vi "Plot Group Config Prompt.vi"(7 "Manager":refnum<class "MessageQ.lvclass">, 9 "Config in":T1, 10 "Init Available Channels":string[](array[string])) -> (1 "Config":T1, 2 "Cancelled":bool)   [LabVIEW 2020, in "VolatusGUIElements.lvlib" / "HistorianCharting.lvclass"]
uses:
  HistorianCharting.lvclass
  VolatusGUI/Historian Charting Manager/X-Axis Type.ctl
  VolatusGUI/Historian Charting Manager/Plot Group Config.ctl
  VolatusGUI/Historian Charting Manager/Plot Config.ctl
  VolatusGUI/Historian Charting Manager/Scale.ctl
  Volatus/MessageQ/MessageQ.lvclass
  lv-autocomplete/AutoComplete/AutoComplete/AutoComplete.lvclass/AutoComplete.ctl
  Volatus/MessageQ/MessageQ.lvclass/MessageQ.ctl
  f20c74bd-5406-41d2-98d9-ce743746d173.vi
  6165f306-330e-4d21-bc48-f8023b5fd340.vi
  c136c978-185a-46ef-8da4-aa5ceb8485eb.vi
  9b52c319-6332-4e64-8368-05bb343efa0c.vi
  lv-autocomplete/AutoComplete/Launch Autocomplete Handler.vi
  <vilib>/Comparison/Less/Less Functor/Less Functor.lvclass
  lv-autocomplete/AutoComplete/AutoComplete/AutoComplete.lvclass
  <vilib>/Comparison/Equal/Equal Functor/Equal Functor.lvclass
  VolatusGUI/Historian Charting Manager/Historian Charting Manager.lvclass
panel:
  out "Group Changes":bool
  in  "X-Axis List":i32(listbox)
  out "Unselected Channels":string[](array[string])
  in  "Dup Group":bool
  in  "X-Axis Channel":string
  in  "Cancel":bool
  in  "Accept":bool
  in  "X-Axis Type":T2
  in  "Remove Group":bool
  in  "New Group":bool
  out "Plot Group":string
  in  "Clear Filter":bool
  in  "Available Channels":i32(listbox)
  in  "Filter":string
  in  "Selected Channels":i32(listbox)
  # "Available Channels"
  # "Double-click to remove channel\nDrag to reorder"
  # "Double-click to add channel"
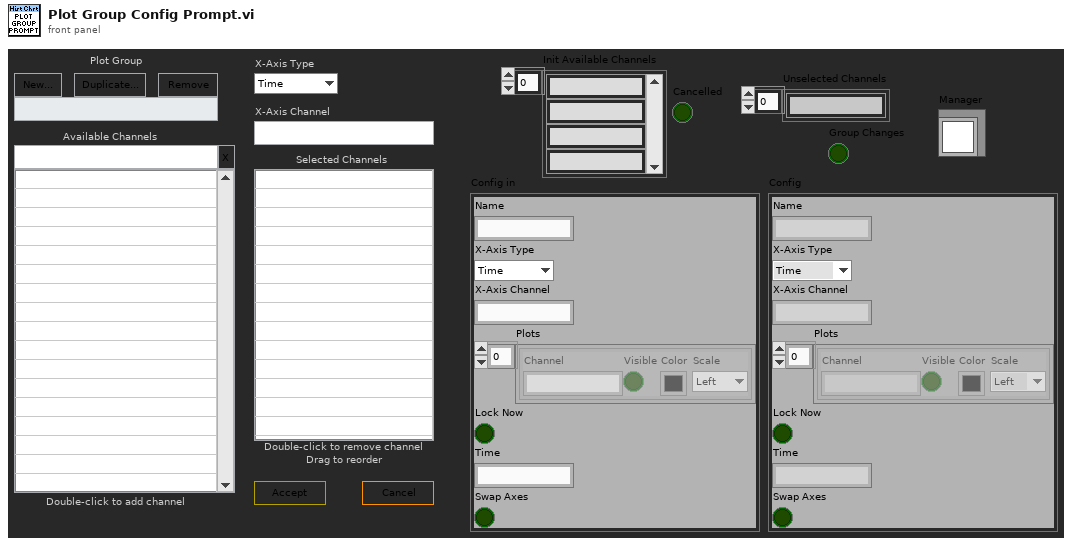
[diagram p1: front panel]
types:
  T1 = typedef "VolatusGUI.lvlib/Historian Charting Manager.lvclass/Plot Group Config.ctl" = cluster{"Name":string, "X-Axis Type":T2, "X-Axis Channel":string, "Plots":T3[], "Lock Now":bool, "Time":string, "Swap Axes":bool}
  T2 = typedef "VolatusGUI.lvlib/Historian Charting Manager.lvclass/X-Axis Type.ctl" = enum16{"Time", "Channel"}
  T3 = typedef "VolatusGUI.lvlib/Historian Charting Manager.lvclass/Plot Config.ctl" = cluster{"Channel":string, "Visible":bool, "Color":u32, "Scale":T4}
  T4 = typedef "VolatusGUI.lvlib/Historian Charting Manager.lvclass/Scale.ctl" = enum16{"Left", "Right"}
  T5 = enum8{"Enabled", "Disabled", "Disabled and Grayed Out"}
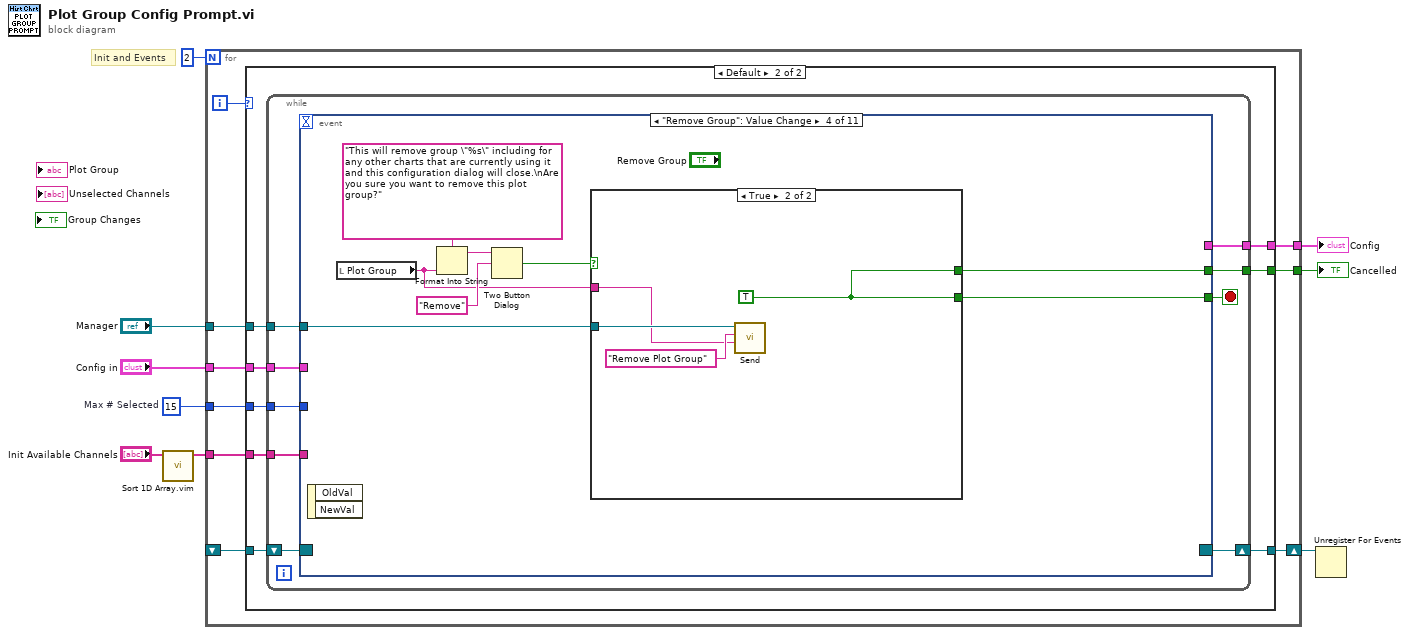
[diagram p0: block diagram]
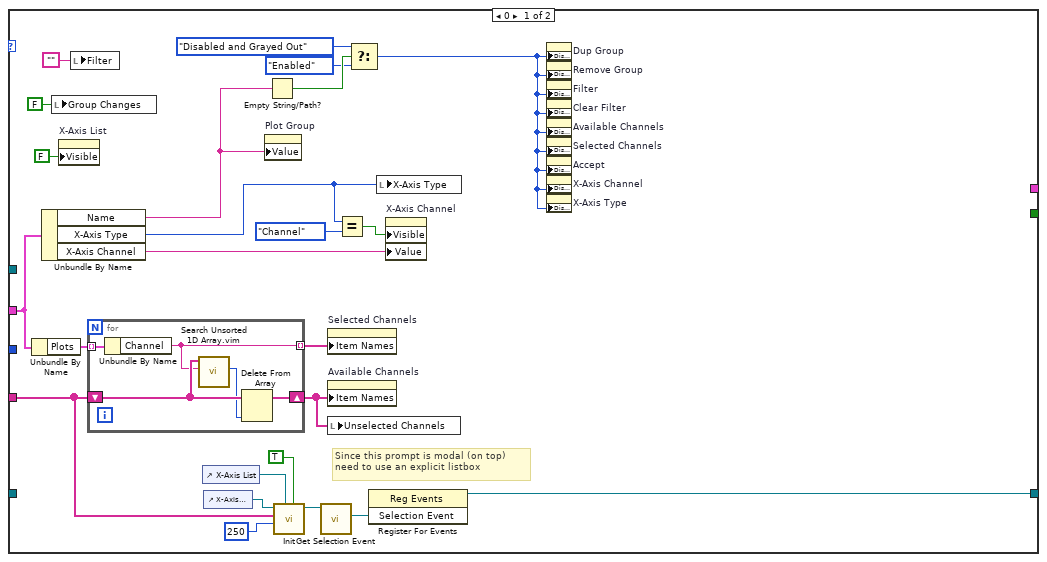
[diagram p2: hidden frame]
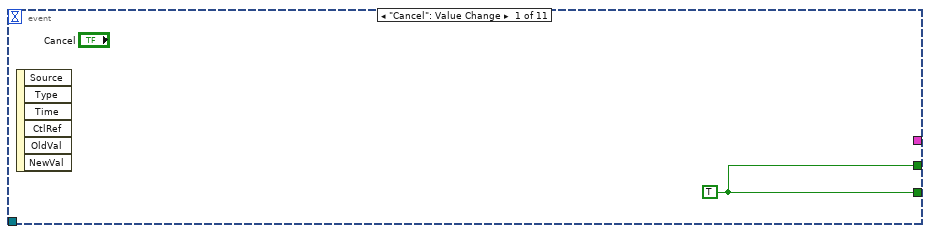
[diagram p3: hidden frame]
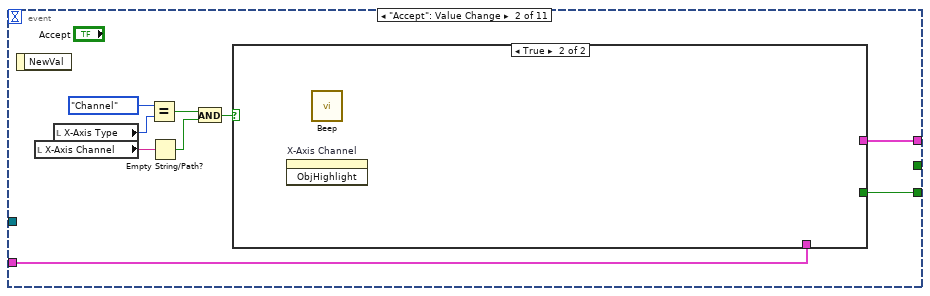
[diagram p4: hidden frame]
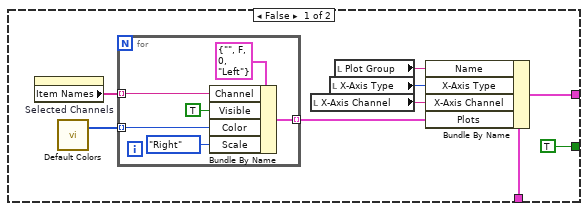
[diagram p5: hidden frame]
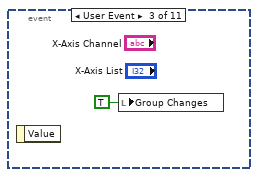
[diagram p6: hidden frame]
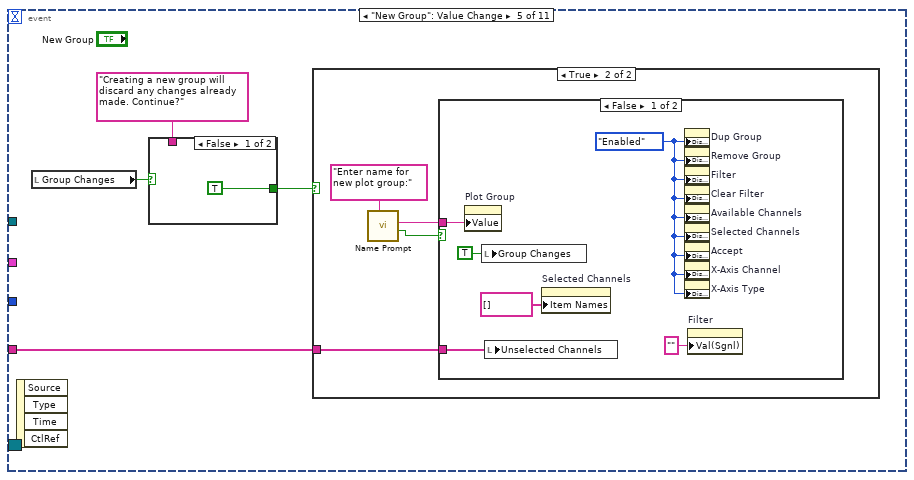
[diagram p8: hidden frame]
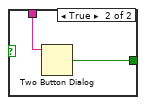
[diagram p11: hidden frame]
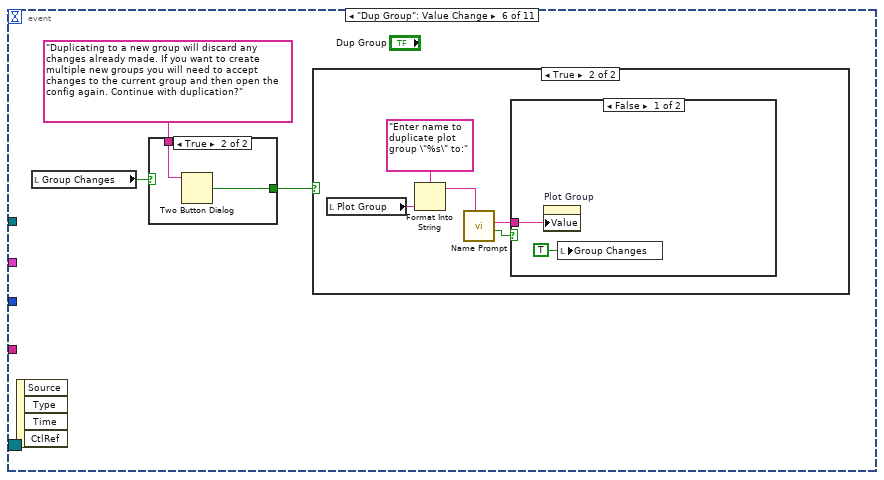
[diagram p12: hidden frame]
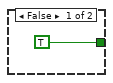
[diagram p15: hidden frame]
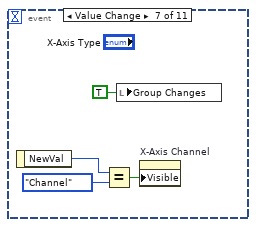
[diagram p16: hidden frame]
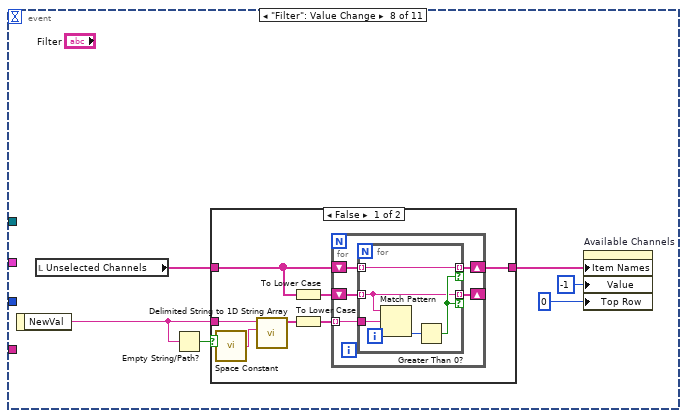
[diagram p17: hidden frame]
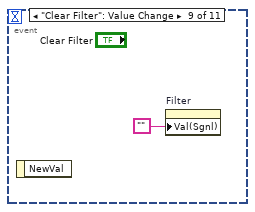
[diagram p19: hidden frame]
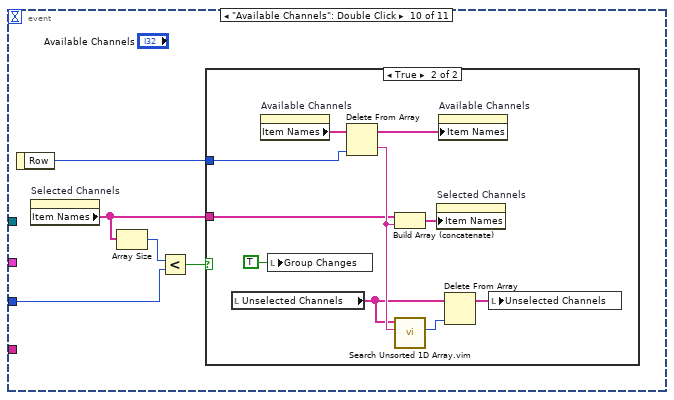
[diagram p20: hidden frame]
diagram:
  w3 = 15  # Max # Selected
  # "Init and Events"
  n1 = call "Sort 1D Array.vim"("unsorted array"="Init Available Channels") -> ("sorted array"=w4:string[])  [unwired: 10 in]
  n2 = for {
    N: 2 -> [_]
    tunnel: [w18] -> w9
    tunnel: w4 -> [w16]
    tunnel: "Config in" -> [w15]
    shift-right: [w14] -> w6
    shift-left: _ -> [w13]
    tunnel: w3 -> [w12]
    tunnel: "Manager" -> [w11]
    tunnel: [w10] -> w1
    i -> [w17]
    n3 = case shown="Default" w17 {
      tunnel: [_ w55] -> w18
      tunnel: w16 -> [w29 w52]
      tunnel: w15 -> [w40 w51]
      tunnel: [w30 w53] -> w14
      tunnel: w13 -> [_ w54]
      tunnel: w12 -> [_ w50]
      tunnel: w11 -> [_ w49]
      tunnel: [_ w48] -> w10
      frame 0 {
        # "Since this prompt is modal (on top) need to use an explicit listbox"
        n4 = Unbundle By Name(w40) -> ("Plots"=w42:T3[])
        n5 = Unbundle By Name(w40) -> ("Name"=w23:string, "X-Axis Type"=w36:T2, "X-Axis Channel"=w39:string)
        n6 = local write "Group Changes"(FALSE ("Group Changes")) -> ()
        n7 = property on="X-Axis List" class="LstBox (strict)"("Visible"=FALSE) -> ()  [unwired: 2 in, 2 out]
        n8 = local write "Filter"("") -> ()
        n9 = for {
          shift-right: [w45] -> w28
          shift-left: w29 -> [w46]
          tunnel: w42 -> [w47] mode=indexing
          tunnel: [w43] -> w41 mode=indexing
          n10 = Unbundle By Name(w47) -> ("Channel"=w43:string)
          n11 = call "Search Unsorted 1D Array.vim"("element"=w43, "unsorted 1D array"=w46) -> ("index of element"=w44:i32)  [unwired: 9 in]
          n12 = Delete From Array(array=w46, index=w44) -> (array with subset deleted=w45:string[])  [unwired: 1 in, 1 out]
        }
        n13 = control-ref of="X-Axis List"() -> (w27:refnum<vi>)
        n14 = control-ref of="X-Axis Channel"() -> (w34:refnum<vi>)
        n15 = property on="Plot Group" class="Str"("Value"=w23) -> ()  [unwired: 2 in, 2 out]
        n16 = Empty String/Path?(string/path=w23) -> (empty?=w21:bool)
        n17 = call "Init.vi"("Autohide ListBox (F)"=TRUE, "ListBox Refnum (Popup)"=w27, "Height (200)"=i16 250, "Initial Options (Empty)"=w29, "Str Refnum"=w34) -> ("AutoComplete out"=w32:refnum<class "AutoComplete.lvclass">)  [unwired: 5 in, 1 out]
        n18 = call "Get Selection Event.vi"("AutoComplete in"=w32) -> ("Selection Event"=w31:refnum<user-event>)  [unwired: 9 in, 1 out]
        n19 = property on="Selected Channels" class="LstBox (strict)"("Item Names"=w41) -> ()  [unwired: 2 in, 2 out]
        n20 = property on="Available Channels" class="LstBox (strict)"("Item Names"=w28) -> ()  [unwired: 2 in, 2 out]
        n21 = local write "Unselected Channels"(w28) -> ()
        n22 = Equal?(x=w36, y=X-Axis_Type."Channel") -> (x = y?=w35:bool)
        n23 = Select(t=T5."Disabled and Grayed Out" ("Disabled"), s=w21, f=T5."Enabled") -> (s? t:f=w19:T5)
        n24 = register-events(w31) -> (reference out=w30:refnum<event-registration>)  [unwired: 2 in, 1 out]
        n25 = local write "X-Axis Type"(w36) -> ()
        n26 = property on="X-Axis Channel" class="Str"("Visible"=w35, "Value"=w39) -> ()  [unwired: 2 in, 2 out]
        n27 = property on="Dup Group" class="Bool"("DisabledEnum"=w19) -> ()  [unwired: 2 in, 2 out]
        n28 = property on="Remove Group" class="Bool"("DisabledEnum"=w19) -> ()  [unwired: 2 in, 2 out]
        n29 = property on="Filter" class="Str"("DisabledEnum"=w19) -> ()  [unwired: 2 in, 2 out]
        n30 = property on="Clear Filter" class="Bool"("DisabledEnum"=w19) -> ()  [unwired: 2 in, 2 out]
        n31 = property on="Available Channels" class="LstBox (strict)"("DisabledEnum"=w19) -> ()  [unwired: 2 in, 2 out]
        n32 = property on="Selected Channels" class="LstBox (strict)"("DisabledEnum"=w19) -> ()  [unwired: 2 in, 2 out]
        n33 = property on="Accept" class="Bool"("DisabledEnum"=w19) -> ()  [unwired: 2 in, 2 out]
        n34 = property on="X-Axis Channel" class="Str"("DisabledEnum"=w19) -> ()  [unwired: 2 in, 2 out]
        n35 = property on="X-Axis Type" class="Enum (strict)"("DisabledEnum"=w19) -> ()  [unwired: 2 in, 2 out]
      }
      frame Default {
        n36 = while {
          tunnel: [w63] -> w55
          shift-right: [w61] -> w53
          shift-left: w54 -> [w62]
          tunnel: w52 -> [w60]
          tunnel: w51 -> [w59]
          tunnel: w50 -> [w58]
          tunnel: w49 -> [w57]
          tunnel: [w56] -> w48
          stop <- w64 stop-if-true
          n37 = event shown="[3] \"Remove Group\": Value Change" {
            selector: w62 -> [_ _ _ _ _ _ _ _ _ _ _]
            dyn-events: [_ _ _ _ _ _ _ _ _ _ _] -> w61
            timeout: _ -> [_ _ _ _ _ _ _ _ _ _ _]
            tunnel: [w65 w67 _ w92 _ _ _ _ _ _ _] -> w64
            tunnel: [w65 _ _ w91 _ _ _ _ _ _ _] -> w63
            tunnel: w60 -> [_ _ _ _ w103 _ _ _ _ _ _]
            tunnel: w59 -> [_ w74 _ _ _ _ _ _ _ _ _]
            tunnel: w58 -> [_ _ _ _ _ _ _ _ _ w163 _]
            tunnel: w57 -> [_ _ _ w94 _ _ _ _ _ _ _]
            tunnel: [_ w73 _ _ _ _ _ _ _ _ _] -> w56
            event "Cancel": Value Change {
              w65 = TRUE
              n38 = event-data() -> ()  [unwired: 1 in, 6 out]
            }
            event "Accept": Value Change {
              n39 = event-data() -> ()  [unwired: 1 in, 1 out]
              n40 = local read "X-Axis Channel"() -> (w70:string)
              n41 = local read "X-Axis Type"() -> (w72:T2)
              n42 = Equal?(x=X-Axis_Type."Channel", y=w72) -> (x = y?=w69:bool)
              n43 = Empty String/Path?(string/path=w70) -> (empty?=w68:bool)
              n44 = And(x=w69, y=w68) -> (x .and. y?=w66:bool)
              n45 = case shown="True" w66 {
                tunnel: w74 -> [w81 _]
                tunnel: [w77 _] -> w73
                tunnel: [TRUE _] -> w67
                frame False {
                  n46 = property on="Selected Channels" class="LstBox (strict)"() -> ("Item Names"=w83:string[])  [unwired: 2 in, 2 out]
                  n47 = call "Default Colors.vi"() -> ("Default Colors"=w82:u32[])  [unwired: 7 in]
                  n48 = for {
                    tunnel: w83 -> [w88] mode=indexing
                    tunnel: w82 -> [w85] mode=indexing
                    tunnel: [w84] -> w80 mode=indexing
                    n49 = Bundle By Name(cluster=T3 {"Channel"="", "Visible"=FALSE, "Color"=0, "Scale"=enum."Left"} ("Plot Config"), "Channel"=w88, "Visible"=TRUE, "Color"=w85, "Scale"=Scale."Right") -> (w84:T3)
                  }
                  n50 = local read "X-Axis Channel"() -> (w78:string)
                  n51 = local read "X-Axis Type"() -> (w79:T2)
                  n52 = local read "Plot Group"() -> (w76:string)
                  n53 = Bundle By Name(cluster=w81, "Name"=w76, "X-Axis Type"=w79, "X-Axis Channel"=w78, "Plots"=w80) -> (w77:T1)
                }
                frame True {
                  n54 = invoke on="X-Axis Channel" class="Str" method="ObjHighlight"() -> ()  [unwired: 3 in, 3 out]
                  n55 = call <vilib>:"Beep.vi"() -> ()  [unwired: 12 in]
                }
              }
            }
            event User Event {
              n56 = event-data() -> ()  [unwired: 1 in, 1 out]
              n57 = local write "Group Changes"(TRUE ("Group Changes")) -> ()
            }
            event "Remove Group": Value Change {
              n58 = event-data() -> ()  [unwired: 1 in, 2 out]
              n59 = local read "Plot Group"() -> (w93:string)
              n60 = Format Into String(format string="This will remove group \"%s\" including for any other charts that are currently using it and this configuration dialog will close.\nAre you sure you want to remove this plot group?", w93) -> (resulting string=w97:string)  [unwired: 2 in, 1 out]
              n61 = Two Button Dialog(message=w97, 2:"Remove" ("T button name (\"OK\")")) -> (T button?=w95:bool)  [unwired: 1 in]
              n62 = case shown="True" w95 {
                tunnel: w94 -> [_ w102]
                tunnel: w93 -> [_ w100]
                tunnel: [_ w99] -> w92
                tunnel: [_ w99] -> w91
                frame False {
                }
                frame True {
                  w99 = TRUE
                  n63 = call "Send.vi"("Data"=w100, "ID"="Remove Plot Group", "MessageQ in"=w102) -> ()  [unwired: 7 in, 2 out]
                }
              }
            }
            event "New Group": Value Change {
              n64 = event-data() -> ()  [unwired: 1 in, 4 out]
              n65 = local read "Group Changes"() -> (w106:bool)
              n66 = case shown="False" w106 {
                tunnel: "Creating a new group will discard any changes already made. Continue?" -> [_ w119]
                tunnel: [TRUE ("T button?") w118] -> w104
                frame False {
                }
                frame True {
                  n67 = Two Button Dialog(message=w119) -> (T button?=w118:bool)  [unwired: 2 in]
                }
              }
              n68 = case shown="True" w104 {
                tunnel: w103 -> [_ w107]
                frame False {
                }
                frame True {
                  n69 = call "Name Prompt.vi"("Prompt"="Enter name for new plot group:") -> ("Cancelled"=w108:bool, "Name"=w110:string)  [unwired: 9 in]
                  n70 = case shown="False" w108 {
                    tunnel: w110 -> [w115 _]
                    tunnel: w107 -> [w112 _]
                    frame False {
                      w114 = T5."Enabled" ("Disabled")
                      n71 = property on="Plot Group" class="Str"("Value"=w115) -> ()  [unwired: 2 in, 2 out]
                      n72 = local write "Group Changes"(TRUE ("Group Changes")) -> ()
                      n73 = local write "Unselected Channels"(w112) -> ()
                      n74 = property on="Selected Channels" class="LstBox (strict)"("Item Names"=string[] []) -> ()  [unwired: 2 in, 2 out]
                      n75 = property on="Dup Group" class="Bool"("DisabledEnum"=w114) -> ()  [unwired: 2 in, 2 out]
                      n76 = property on="Remove Group" class="Bool"("DisabledEnum"=w114) -> ()  [unwired: 2 in, 2 out]
                      n77 = property on="Filter" class="Str"("DisabledEnum"=w114) -> ()  [unwired: 2 in, 2 out]
                      n78 = property on="Clear Filter" class="Bool"("DisabledEnum"=w114) -> ()  [unwired: 2 in, 2 out]
                      n79 = property on="Available Channels" class="LstBox (strict)"("DisabledEnum"=w114) -> ()  [unwired: 2 in, 2 out]
                      n80 = property on="Selected Channels" class="LstBox (strict)"("DisabledEnum"=w114) -> ()  [unwired: 2 in, 2 out]
                      n81 = property on="Accept" class="Bool"("DisabledEnum"=w114) -> ()  [unwired: 2 in, 2 out]
                      n82 = property on="X-Axis Channel" class="Str"("DisabledEnum"=w114) -> ()  [unwired: 2 in, 2 out]
                      n83 = property on="X-Axis Type" class="Enum (strict)"("DisabledEnum"=w114) -> ()  [unwired: 2 in, 2 out]
                      n84 = property on="Filter" class="Str"("Val(Sgnl)"="" ("Value (Signaling)")) -> ()  [unwired: 2 in, 2 out]
                    }
                    frame True {
                    }
                  }
                }
              }
            }
            event "Dup Group": Value Change {
              n85 = event-data() -> ()  [unwired: 1 in, 4 out]
              n86 = local read "Group Changes"() -> (w122:bool)
              n87 = case shown="True" w122 {
                tunnel: "Duplicating to a new group will discard any changes already made. If you want to create multiple new groups you will need to accept changes to the current group and then open the config again. Continue with duplication?" -> [_ w132]
                tunnel: [TRUE ("T button?") w131] -> w120
                frame False {
                }
                frame True {
                  n88 = Two Button Dialog(message=w132) -> (T button?=w131:bool)  [unwired: 2 in]
                }
              }
              n89 = case shown="True" w120 {
                frame False {
                }
                frame True {
                  n90 = local read "Plot Group"() -> (w125:string)
                  n91 = Format Into String(format string="Enter name to duplicate plot group \"%s\" to:" ("Prompt"), w125) -> (resulting string=w124:string)  [unwired: 2 in, 1 out]
                  n92 = call "Name Prompt.vi"("Prompt"=w124) -> ("Cancelled"=w126:bool, "Name"=w127:string)  [unwired: 9 in]
                  n93 = case shown="False" w126 {
                    tunnel: w127 -> [w129 _]
                    frame False {
                      n94 = property on="Plot Group" class="Str"("Value"=w129) -> ()  [unwired: 2 in, 2 out]
                      n95 = local write "Group Changes"(TRUE ("Group Changes")) -> ()
                    }
                    frame True {
                    }
                  }
                }
              }
            }
            event Value Change {
              n96 = event-data() -> ("NewVal"=w136:T2)  [unwired: 1 in]
              n97 = Equal?(x=w136, y=X-Axis_Type."Channel") -> (x = y?=w134:bool)
              n98 = local write "Group Changes"(TRUE ("Group Changes")) -> ()
              n99 = property on="X-Axis Channel" class="Str"("Visible"=w134) -> ()  [unwired: 2 in, 2 out]
            }
            event "Filter": Value Change {
              n100 = event-data() -> ("NewVal"=w138:string)  [unwired: 1 in]
              n101 = local read "Unselected Channels"() -> (w142:string[])
              n102 = Empty String/Path?(string/path=w138) -> (empty?=w137:bool)
              n103 = case shown="False" w137 {
                tunnel: w138 -> [w149 _]
                tunnel: w142 -> [w145 w160]
                tunnel: [w143 w160] -> w141
                frame False {
                  n104 = call <vilib>:"Space Constant.vi"() -> ("String"=w148:string)
                  n105 = call <vilib>:"Delimited String to 1D String Array.vi"("delimiter"=w148, "delimited string"=w149) -> ("string array"=w147:string[])  [unwired: 9 in]
                  n106 = To Lower Case(string=w145) -> (all lower case string=w144:string[])
                  n107 = To Lower Case(string=w147) -> (all lower case string=w146:string[])
                  n108 = for {
                    shift-right: [w153] -> w143
                    shift-left: w145 -> [w152]
                    tunnel: w146 -> [w154] mode=indexing
                    shift-right: [w150] -> _
                    shift-left: w144 -> [w151]
                    n109 = for {
                      tunnel: w154 -> [w158]
                      tunnel: [w159] -> w153 mode=indexing if=w156
                      tunnel: w152 -> [w159] mode=indexing
                      tunnel: w151 -> [w155] mode=indexing
                      tunnel: [w155] -> w150 mode=indexing if=w156
                      n110 = Match Pattern(string=w155, regular expression=w158) -> (offset past match=w157:i32)  [unwired: 1 in, 3 out]
                      n111 = Greater Than 0?(x=w157) -> (x > 0?=w156:bool)
                    }
                  }
                }
                frame True {
                }
              }
              n112 = property on="Available Channels" class="LstBox (strict)"("Item Names"=w141, "Value"=-1 ("Available Channels"), "Top Row"=0) -> ()  [unwired: 2 in, 2 out]
            }
            event "Clear Filter": Value Change {
              n113 = event-data() -> ()  [unwired: 1 in, 1 out]
              n114 = property on="Filter" class="Str"("Val(Sgnl)"="") -> ()  [unwired: 2 in, 2 out]
            }
            event "Available Channels": Double Click {
              n115 = event-data() -> ("Row"=w166:i32)  [unwired: 1 in]
              n116 = property on="Selected Channels" class="LstBox (strict)"() -> ("Item Names"=w165:string[])  [unwired: 2 in, 2 out]
              n117 = Array Size(array=w165) -> (size(s)=w164:i32)
              n118 = Less?(x=w164, y=w163) -> (x < y?=w162:bool)
              n119 = case shown="True" w162 {
                tunnel: w166 -> [_ w175]
                tunnel: w165 -> [_ w168]
                frame False {
                  n120 = call <vilib>:"Beep.vi"() -> ()  [unwired: 12 in]
                  n121 = invoke on="Selected Channels" class="LstBox (strict)" method="ObjHighlight"() -> ()  [unwired: 3 in, 3 out]
                }
                frame True {
                  n122 = local read "Unselected Channels"() -> (w171:string[])
                  n123 = property on="Available Channels" class="LstBox (strict)"() -> ("Item Names"=w176:string[])  [unwired: 2 in, 2 out]
                  n124 = local write "Group Changes"(TRUE ("Group Changes")) -> ()
                  n125 = Delete From Array(array=w176, index=w175) -> (deleted portion=w172:string, array with subset deleted=w174:string[])  [unwired: 1 in]
                  n126 = Build Array (concatenate)(w168, w172) -> (w173:string[])
                  n127 = call "Search Unsorted 1D Array.vim"("element"=w172, "unsorted 1D array"=w171) -> ("index of element"=w170:i32)  [unwired: 9 in]
                  n128 = property on="Selected Channels" class="LstBox (strict)"("Item Names"=w173) -> ()  [unwired: 2 in, 2 out]
                  n129 = property on="Available Channels" class="LstBox (strict)"("Item Names"=w174) -> ()  [unwired: 2 in, 2 out]
                  n130 = Delete From Array(array=w171, index=w170) -> (array with subset deleted=w169:string[])  [unwired: 1 in, 1 out]
                  n131 = local write "Unselected Channels"(w169) -> ()
                }
              }
            }
            event "Selected Channels": Double Click {
              n132 = event-data() -> ("Row"=w185:i32)  [unwired: 1 in]
              n133 = local read "Unselected Channels"() -> (w182:string[])
              n134 = property on="Selected Channels" class="LstBox (strict)"() -> ("Item Names"=w186:string[])  [unwired: 2 in, 2 out]
              n135 = local read "Filter"() -> (w178:string)
              n136 = Delete From Array(array=w186, index=w185) -> (deleted portion=w181:string, array with subset deleted=w184:string[])  [unwired: 1 in]
              n137 = property on="Filter" class="Str"("Val(Sgnl)"=w178) -> ()  [unwired: 2 in, 2 out]
              n138 = Build Array (concatenate)(w182, w181) -> (w180:string[])
              n139 = property on="Selected Channels" class="LstBox (strict)"("Item Names"=w184, "Value"=-1 ("Selected Channels")) -> ()  [unwired: 2 in, 2 out]
              n140 = call "Sort 1D Array.vim"("unsorted array"=w180) -> ("sorted array"=w179:string[])  [unwired: 10 in]
              n141 = local write "Unselected Channels"(w179) -> ()
              n142 = local write "Group Changes"(TRUE ("Group Changes")) -> ()
            }
          }
        }
      }
    }
  }
  "Config" <- w1
  "Cancelled" <- w9
  n143 = Unregister For Events(event registration refnum=w6) -> ()  [unwired: 1 in, 1 out]
